vi "check if root actor.vi"(11 "Template in":refnum<class "Template.lvclass">) -> (3 "Is Root Actor?":bool)   [LabVIEW 2020, in "Template.lvlib" / "Template.lvclass"]
doc: "Returns True if this is the root actor"
uses:
  Template.lvclass
  C:/Program Files/National Instruments/LabVIEW 2020/vi.lib/ActorFramework/Actor/Actor.lvclass
  <vilib>/ActorFramework/Actor/Actor.lvclass/Actor.ctl
  <vilib>/ActorFramework/Message Enqueuer/Message Enqueuer.lvclass
  Template.lvclass/Template.ctl
  <vilib>/ActorFramework/Actor/Actor.lvclass
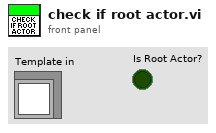
[diagram p1: front panel]
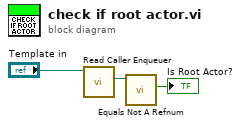
[diagram p0: block diagram]
diagram:
  n1 = call <vilib>:"Read Caller Enqueuer.vi"("Actor"="Template in") -> ("Caller Enqueuer"=w2:refnum<class "Message Enqueuer.lvclass">)  [unwired: 10 in]
  n2 = call <vilib>:"Equals Not A Refnum.vi"("Message Enqueuer"=w2) -> ("Not a refnum?"=→"Is Root Actor?":bool)  [unwired: 10 in]
